vi "Correct_root_path.vi"(7 "Display warning? (T)":bool=TRUE, 8 "error in (no error)":errorcluster) -> (0 "error out":errorcluster, 2 "Path is correct?":bool, 3 "Resulting path":path)   [LabVIEW 2017]
uses:
  <vilib>/Utility/sysdir.llb/System Directory Type.ctl
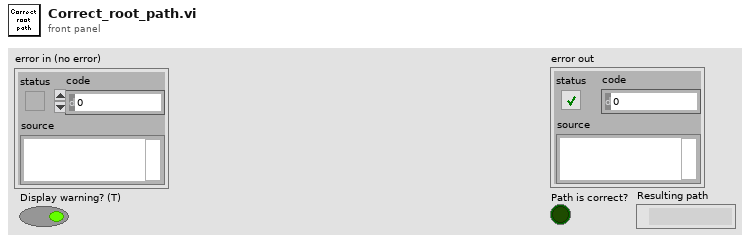
[diagram p1: front panel]
types:
  T1 = typedef "System Directory Type.ctl" = i32
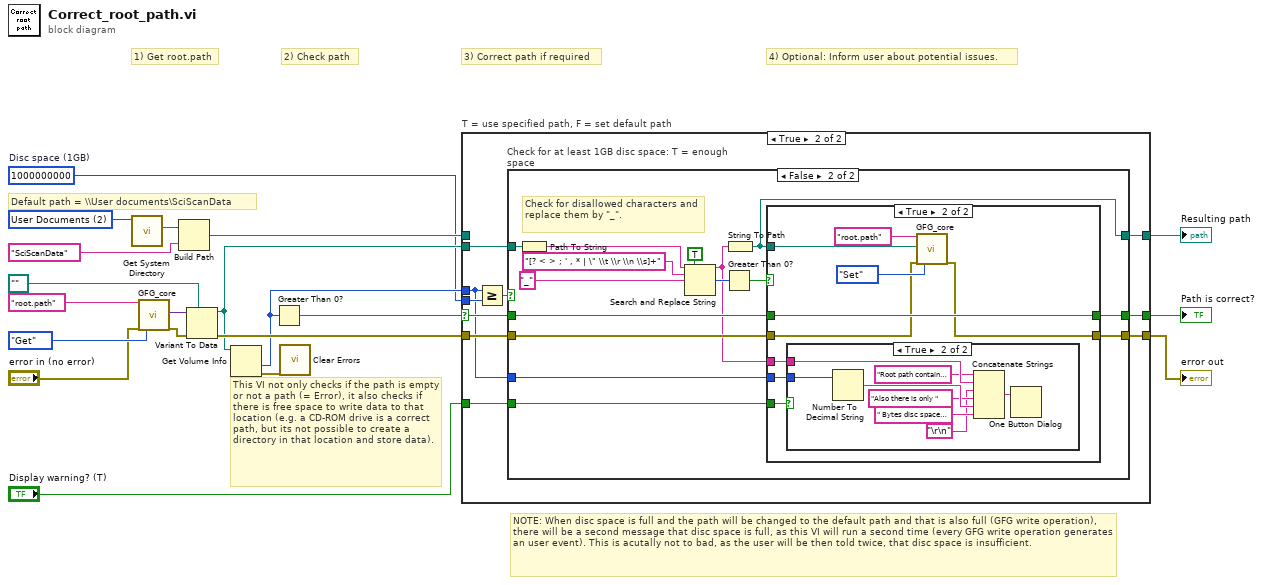
[diagram p0: block diagram]
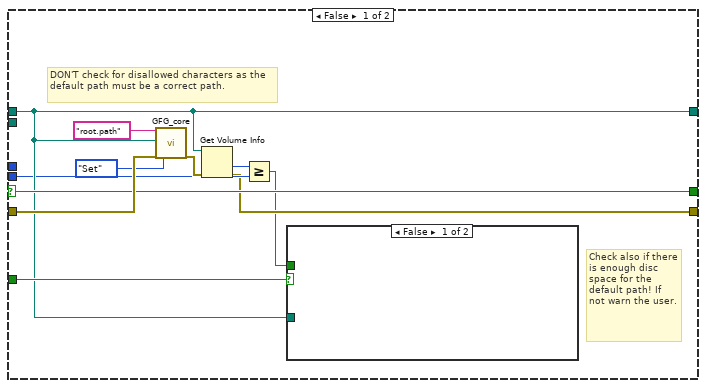
[diagram p2: hidden frame]
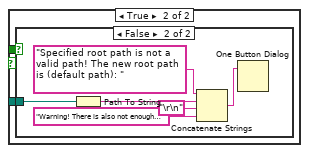
[diagram p3: hidden frame]
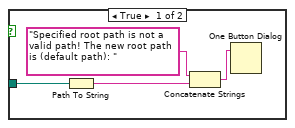
[diagram p4: hidden frame]
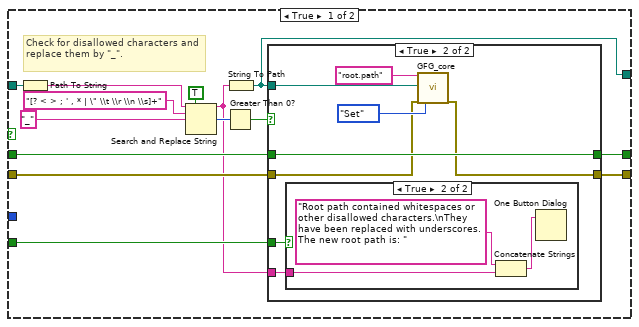
[diagram p5: hidden frame]
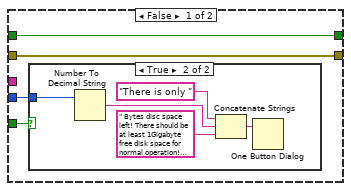
[diagram p8: hidden frame]
diagram:
  w1 = i64 1000000000  # Disc space (1GB)
  w7 = T1 2 items=["User Home"=0, "User Desktop"=1, "User Documents"=2, "User Application Data"=3, "User Preferences"=4, "User Temporary"=5, "Public Documents"=6, "Public Application Data"=7, "Public Preferences"=8, "Public Cache"=13, "System Core Libraries"=9, "System Installed Libraries"=10, "Application Files"=11, "Boot Volume Root"=12] ("system directory type")
  # "NOTE: When disc space is full and the path will be changed to the default path and that is also full (GFG write operation), there will be a second message that disc space is full, as this VI will run a second time (every GFG write operation generates an user event). This is acutally not to bad, as the user will be then told twice, that disc space is insufficient."
  # "4) Optional: Inform user about potential issues."
  # "Default path = \\\\User documents\\SciScanData"
  # "1) Get root.path"
  # "This VI not only checks if the path is empty or not a path (= Error), it also checks if there is free space to write data to that location (e.g. a CD-ROM drive is a correct path, but its not possible to create a directory in that location and store data)."
  # "3) Correct path if required"
  # "2) Check path"
  n1 = call <vilib>:"Get System Directory.vi"("system directory type"=w7) -> ("system directory"=w6:path)  [unwired: 10 in]
  n2 = call "GFG_core.vi"("Variable Name in"="root.path", "error in (no error)"="error in (no error)", "Action"=enum16{"Init", "Set", "Get", "Clear"}."Get") -> ("Variant Out"=w12:variant, "error out"=w13:errorcluster)  [unwired: 10 in, 5 out]
  n3 = Build Path(base path=w6, name or relative path="SciScanData") -> (appended path=w4:path)
  n4 = Variant To Data(error in=w13, type=path "" ("path"), Variant=w12) -> (data=w8:path, error out=w19:errorcluster)
  n5 = Get Volume Info(11:w8) -> (0:w18:errorcluster, 1:w2:i64)  [unwired: 1 in, 4 out]
  n6 = Greater Than 0?(x=w2) -> (x > 0?=w3:bool)
  n7 = call <vilib>:"Clear Errors.vi"("error in (no error)"=w18) -> ()  [unwired: 5 in, 2 out]
  n8 = case "T = use specified path, F = set default path" shown="True" w3 {
    selector: w3 -> [w29 w52]
    tunnel: w4 -> [w25 _]
    tunnel: w19 -> [w31 w49]
    tunnel: [w22 w48] -> w20
    tunnel: [w25 w50] -> w17
    tunnel: [w29 w51] -> w16
    tunnel: "Display warning? (T)" -> [w30 w47]
    tunnel: w8 -> [_ w53]
    tunnel: w2 -> [_ w44]
    tunnel: w1 -> [w23 w46]
    frame False {
      # "Check also if there is enough disc space for the default path! If not warn the user."
      # "DON'T check for disallowed characters as the default path must be a correct path."
      n9 = call "GFG_core.vi"("Variable Name in"="root.path", "Variant in"=w25, "error in (no error)"=w31, "Action"=enum16{"Init", "Set", "Get", "Clear"}."Set") -> ("error out"=w26:errorcluster)  [unwired: 9 in, 6 out]
      n10 = Get Volume Info(8:w26, 11:w25) -> (0:w22:errorcluster, 1:w24:i64)  [unwired: 4 out]
      n11 = Greater Or Equal?(x=w24, y=w23) -> (x >= y?=w21:bool)
      n12 = case shown="False" w30 {
        tunnel: w25 -> [_ w33]
        tunnel: w21 -> [_ w32]
        frame False {
        }
        frame True {
          n13 = case shown="False" w32 {
            tunnel: w33 -> [w37 w43]
            frame True {
              n14 = Path To String(path=w37) -> (string=w36:string)
              n15 = Concatenate Strings("Specified root path is not a valid path! The new root path is (default path): " ("message"), w36) -> (w34:string)
              n16 = One Button Dialog(message=w34) -> ()  [unwired: 1 in, 1 out]
            }
            frame False {
              n17 = Path To String(path=w43) -> (string=w42:string)
              n18 = Concatenate Strings("Specified root path is not a valid path! The new root path is (default path): " ("message"), w42, "\r\n", "Warning! There is also not enough disc space using the default path. Free disc space, otherwise data will be lost." ("message")) -> (w40:string)
              n19 = One Button Dialog(message=w40) -> ()  [unwired: 1 in, 1 out]
            }
          }
        }
      }
    }
    frame True {
      n20 = Greater Or Equal?(x=w44, y=w46) -> (x >= y?=w45:bool)
      n21 = case "Check for at least 1GB disc space: T = enough space" shown="False" w45 {
        tunnel: w53 -> [w63 w91]
        tunnel: w52 -> [w60 w88]
        tunnel: [w59 w87] -> w51
        tunnel: [w58 w86] -> w50
        tunnel: w49 -> [w57 w85]
        tunnel: [w56 w84] -> w48
        tunnel: w47 -> [w55 w83]
        tunnel: w44 -> [_ w82]
        frame True {
          # "Check for disallowed characters and replace them by \"_\"."
          n22 = Path To String(path=w63) -> (string=w64:string)
          n23 = Search and Replace String(replace all?=TRUE ("replace all? (F)"), input string=w64, search string="[? < > ; ' , * | \" \\t \\r \\n \\s]+", replace string="_" ("replace string (\"\")")) -> (result string=w54:string, number of replacements=w62:i32)  [unwired: 4 in, 2 out]
          n24 = Greater Than 0?(x=w62) -> (x > 0?=w61:bool)
          n25 = String To Path(string=w54) -> (path=w58:path)
          n26 = case shown="True" w61 {
            tunnel: w58 -> [_ w75]
            tunnel: w60 -> [w69 w74]
            tunnel: [w69 w74] -> w59
            tunnel: w57 -> [w68 w73]
            tunnel: [w68 w72] -> w56
            tunnel: w55 -> [_ w71]
            tunnel: w54 -> [_ w70]
            frame False {
            }
            frame True {
              n27 = case shown="True" w71 {
                tunnel: w70 -> [_ w78]
                frame False {
                }
                frame True {
                  n28 = Concatenate Strings("Root path contained whitespaces or other disallowed characters.\nThey have been replaced with underscores. The new root path is: ", w78) -> (w80:string)
                  n29 = One Button Dialog(message=w80) -> ()  [unwired: 1 in, 1 out]
                }
              }
              n30 = call "GFG_core.vi"("Variable Name in"="root.path", "Variant in"=w75, "error in (no error)"=w73, "Action"=enum16{"Init", "Set", "Get", "Clear"}."Set") -> ("error out"=w72:errorcluster)  [unwired: 9 in, 6 out]
            }
          }
        }
        frame False {
          # "Check for disallowed characters and replace them by \"_\"."
          n31 = Path To String(path=w91) -> (string=w92:string)
          n32 = Search and Replace String(replace all?=TRUE ("replace all? (F)"), input string=w92, search string="[? < > ; ' , * | \" \\t \\r \\n \\s]+", replace string="_" ("replace string (\"\")")) -> (result string=w81:string, number of replacements=w90:i32)  [unwired: 4 in, 2 out]
          n33 = Greater Than 0?(x=w90) -> (x > 0?=w89:bool)
          n34 = String To Path(string=w81) -> (path=w86:path)
          n35 = case shown="True" w89 {
            tunnel: w86 -> [_ w111]
            tunnel: w88 -> [w99 w110]
            tunnel: [w99 w110] -> w87
            tunnel: w85 -> [w98 w109]
            tunnel: [w98 w108] -> w84
            tunnel: w83 -> [w97 w107]
            tunnel: w82 -> [w96 w106]
            tunnel: w81 -> [_ w105]
            frame False {
              n36 = case shown="True" w97 {
                tunnel: w96 -> [_ w100]
                frame False {
                }
                frame True {
                  n37 = Number To Decimal String(number=w100) -> (decimal integer string=w103:string)  [unwired: 1 in]
                  n38 = Concatenate Strings("There is only " ("message"), w103, " Bytes disc space left! There should be at least 1Gigabyte free disk space for normal operation! Free disc space or use another path, otherwise data will be lost." ("message")) -> (w102:string)
                  n39 = One Button Dialog(message=w102) -> ()  [unwired: 1 in, 1 out]
                }
              }
            }
            frame True {
              n40 = case shown="True" w107 {
                tunnel: w106 -> [_ w117]
                tunnel: w105 -> [_ w115]
                frame False {
                }
                frame True {
                  n41 = Number To Decimal String(number=w117) -> (decimal integer string=w120:string)  [unwired: 1 in]
                  n42 = Concatenate Strings("Root path contained whitespaces or other disallowed characters.\nThey have been replaced with underscores. The new root path is: ", w115, "\r\n", "Also there is only " ("message"), w120, " Bytes disc space left! There should be at least 1Gigabyte free disk space for normal operation! Free disc space or use another path, otherwise data will be lost." ("message")) -> (w119:string)
                  n43 = One Button Dialog(message=w119) -> ()  [unwired: 1 in, 1 out]
                }
              }
              n44 = call "GFG_core.vi"("Variable Name in"="root.path", "Variant in"=w111, "error in (no error)"=w109, "Action"=enum16{"Init", "Set", "Get", "Clear"}."Set") -> ("error out"=w108:errorcluster)  [unwired: 9 in, 6 out]
            }
          }
        }
      }
    }
  }
  "error out" <- w20
  "Path is correct?" <- w16
  "Resulting path" <- w17
